vi "Measurement.vi"(8 "error in (no error)":errorcluster, 11 "IV in":refnum<class "IV.lvclass">) -> (0 "error out":errorcluster, 1 "Finish?":bool, 2 "Result":dbl, 3 "IV out":refnum<class "IV.lvclass">)   [LabVIEW 2018, in "IV.lvclass"]
uses:
  IV.lvclass
  Experiment/Experiment2D/Experiment2D.lvclass
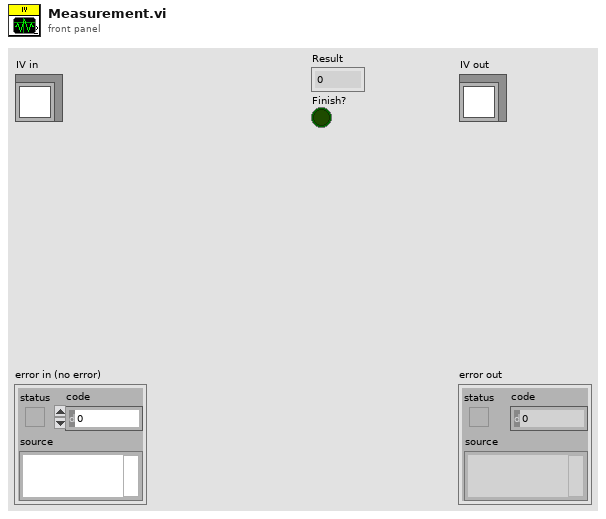
[diagram p1: front panel]
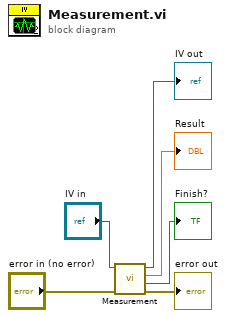
[diagram p0: block diagram]
diagram:
  n1 = call-parent "Measurement.vi"("error in (no error)"="error in (no error)", "Experiment2D in"="IV in") -> ("error out"=→"error out":errorcluster, "Finish?"=→"Finish?":bool, "Result"=→"Result":dbl, "Experiment2D out"=→"IV out":refnum<class "IV.lvclass">)  [unwired: 6 in]
